vi "run.vi"(8 "error in (no error)":errorcluster, 10 "Path":path, 11 "ICSettingsViewer in":refnum<class "ICSettingsViewer.lvclass">) -> (0 "error out":errorcluster, 3 "ICSettingsViewer out":refnum<class "ICSettingsViewer.lvclass">)   [LabVIEW 2011, in "Views.lvlib" / "Camera.lvlib" / "ICSettingsViewer.lvclass"]
uses:
  ICSettingsViewer.lvclass
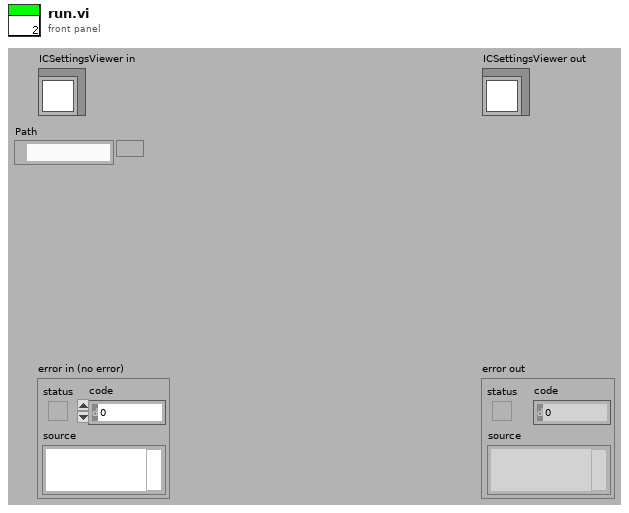
[diagram p1: front panel]
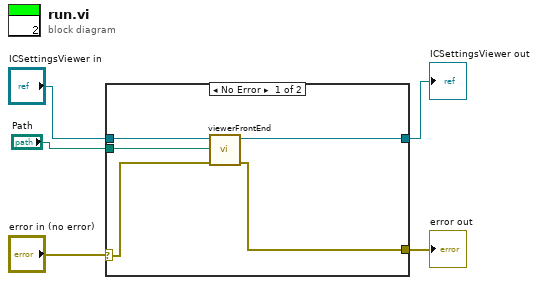
[diagram p0: block diagram]
diagram:
  n1 = case shown="No Error" "error in (no error)" {
    selector: "error in (no error)" -> [w7 w11]
    tunnel: "ICSettingsViewer in" -> [w10 w12]
    tunnel: "Path" -> [w9 _]
    tunnel: [w8 w12] -> w2
    tunnel: [w6 w11] -> w1
    frame No Error {
      n2 = call-dynamic "viewerFrontEnd.vi"("error in (no error)"=w7, "defaultPath"=w9, "ICSettingsViewer in"=w10) -> ("error out"=w6:errorcluster, "ICSettingsViewer out"=w8:refnum<class "ICSettingsViewer.lvclass">)  [unwired: 7 in]
    }
    frame Error {
    }
  }
  "error out" <- w1
  "ICSettingsViewer out" <- w2
